vi "Permanentes_Aux.vi"() -> ()   [LabVIEW 2013]
uses:
  <vilib>/Utility/miscctls.llb/LVStringsAndValuesArrayTypeDef_U16.ctl
panel:
  in  "Puerto COM":refnum<visa-resource-name>
  out "Recetas":T1
  in  "Programa":u16(ring)
  in  "Recetas Allen Bradley":T2(array[cluster]) {"Parámetros Modbus"."Acción al desconectar" items=["Alarmar"=0, "Nada"=3]; "Parámetros Modbus"."Timeout" format="%#_g seg."; "Parámetros Modbus"."Formato de mensaje" items=["8-N-1", "8-E-1", "8-O-1", "8-N-2", "8-E-2", "8-O-2"]; "Parámetros Modbus"."Velocidad" items=["1200 baudios", "2400 baudios", "4800 baudios", "9600 baudios", "19200 baudios", "38400 baudios"]; "Parámetros Modbus"."Identificador" min=1 max=255; "Parámetros Modbus"."Frecuencia estándar" format="%.0fHz."; "Características del motor"."Frecuencia máxima" max=500 format="%.0f Hz."; "Características del motor"."Frecuencia mínima" max=500 format="%.0f Hz."; "Características del motor"."Desaceleración" format="%#_g seg."; "Características del motor"."Aceleración" format="%#_g seg."; "Características del motor"."Velocidad nomial" min=0.0 max=24000.0 format="%#_g rpm"; "Características del motor"."Número de polos" min=2 max=40 format="%.0f polos"; "Características del motor"."Corriente nominal" format="%#_g Amp."; "Características del motor"."Corriente sobrecarga" format="%#_g Amp."; "Características del motor"."Frecuencia nominal" min=15 max=500 format="%.0f Hz."; "Características del motor"."Voltaje nominal" min=20.0 max=440.0 format="%#_g V"; "I/O"."Relevador (R)" items=["Listo/Fallo"=0, "Modbus"=13]; "I/O"."Entrada 6 (06)" items=["Sin asignar"=0, "Fallo auxiliar"=12, "Reset"=13]; "I/O"."Entrada 5 (05)" items=["Sin asignar"=0, "Fallo auxiliar"=12, "Reset"=13]; "I/O"."Entrada 3 (03)" items=["Sin asignar"=0, "Fallo auxiliar"=12, "Reset"=13, "2 hilos REV"=50, "3 hilos DIR"=51]; "I/O"."Entrada 2 (02)" items=["Sin asignar"=0, "Fallo auxiliar"=12, "Reset"=13, "2 hilos FWD"=48, "3 hilos RUN"=49]; "Referencias"."Referencia de frecuencia 2" items=["Potenciómetro"=0, "Modbus"=2]; "Referencias"."Referencia de arranque 2" items=["Teclado", "Pulso", "Modbus"]; "Referencias"."Referencia de frecuencia 1" items=["Potenciómetro"=0, "Modbus"=2]; "Referencias"."Referencia de arranque 1" items=["Teclado", "Pulso", "Modbus"]}
  in  "Recetas Schneider":T3(array[cluster]) {"Parámetros Modbus"."Acción al desconectar" items=["Nada", "Alarmar"]; "Parámetros Modbus"."Timeout" format="%#_g seg."; "Parámetros Modbus"."Formato de mensaje" items=["No", "Auto", "8-O-1", "8-E-1", "8-N-1", "8-N-2", "7-O-1", "7-E-1", "7-O-2", "7-E-2"]; "Parámetros Modbus"."Velocidad" items=["No"=0, "4800 baudios"=24, "9600 baudios"=28, "19200 baudios"=32, "38400 baudios"=36]; "Parámetros Modbus"."Identificador" min=1 max=255; "Parámetros Modbus"."Frecuencia estándar" format="%.0fHz."; "Características del motor"."Desaceleración" format="%#_g seg."; "Características del motor"."Aceleración" format="%#_g seg."; "Características del motor"."Frecuencia máxima" format="%#_g Hz."; "Características del motor"."Velocidad nominal" format="%.0f rpm"; "Características del motor"."Frecuencia nominal" format="%#_g Hz."; "Características del motor"."Corriente nominal" format="%#_g Amp."; "Características del motor"."Voltaje nominal" format="%.0f V"; "Características del motor"."Potencia nominal" format="%#_g HP"; "Características del motor"."Frecuencia estándar" items=["50 Hz.", "60 Hz."]; "I/O"."Transistor (DQ)" items=["Modbus", "Sin Fallo", "Run", "Frecuencia alcanzada", "V. Máx. Alcanzada"]; "I/O"."Relevador 2" items=["Modbus", "Sin Fallo", "Run", "Frecuencia alcanzada", "V. Máx. Alcanzada"]; "I/O"."Relevador 1" items=["Modbus", "Sin Fallo", "Run", "Frecuencia alcanzada", "V. Máx. Alcanzada"]; "I/O"."Entrada 6 (DI6)" items=["Sin asignar"=0, "Marcha"=1, "Marcha av."=2, "Marcha atr."=3, "Referencia 1 Fr."=96, "Referencia 2 Fr."=97, "Referencia 1 Run"=98, "Referencia 2 Run"=99]; "I/O"."Entrada 5 (DI5)" items=["Sin asignar"=0, "Marcha"=1, "Marcha av."=2, "Marcha atr."=3, "Referencia 1 Fr."=96, "Referencia 2 Fr."=97, "Referencia 1 Run"=98, "Referencia 2 Run"=99]; "I/O"."Entrada 4 (DI4)" items=["Sin asignar"=0, "Marcha"=1, "Marcha av."=2, "Marcha atr."=3, "Referencia 1 Fr."=96, "Referencia 2 Fr."=97, "Referencia 1 Run"=98, "Referencia 2 Run"=99]; "I/O"."Entrada 3 (DI3)" items=["Sin asignar"=0, "Marcha"=1, "Marcha av."=2, "Marcha atr."=3, "Referencia 1 Fr."=96, "Referencia 2 Fr."=97, "Referencia 1 Run"=98, "Referencia 2 Run"=99]; "I/O"."Entrada 2 (DI2)" items=["Sin asignar"=0, "Marcha"=1, "Marcha av."=30, "Marcha atr."=31, "Referencia 1 Fr."=96, "Referencia 2 Fr."=97, "Referencia 1 Run"=98, "Referencia 2 Run"=99]; "I/O"."Entrada 1 (DI1)" items=["Sin asignar"=0, "Marcha"=1, "Marcha av."=30, "Marcha atr."=31, "Referencia 1 Fr."=96, "Referencia 2 Fr."=97, "Referencia 1 Run"=98, "Referencia 2 Run"=99]; "Referencias"."Referencia de frecuencia 2" items=["No"=0, "Modbus"=164, "Potenciómetro"=183]; "Referencias"."Referencia de arranque 2" items=["Pulso"=0, "Modbus"=9]; "Referencias"."Referencia de frecuencia 1" items=["No"=0, "Modbus"=164, "Potenciómetro"=183]; "Referencias"."Referencia de arranque 1" items=["Pulso"=0, "Modbus"=9]}
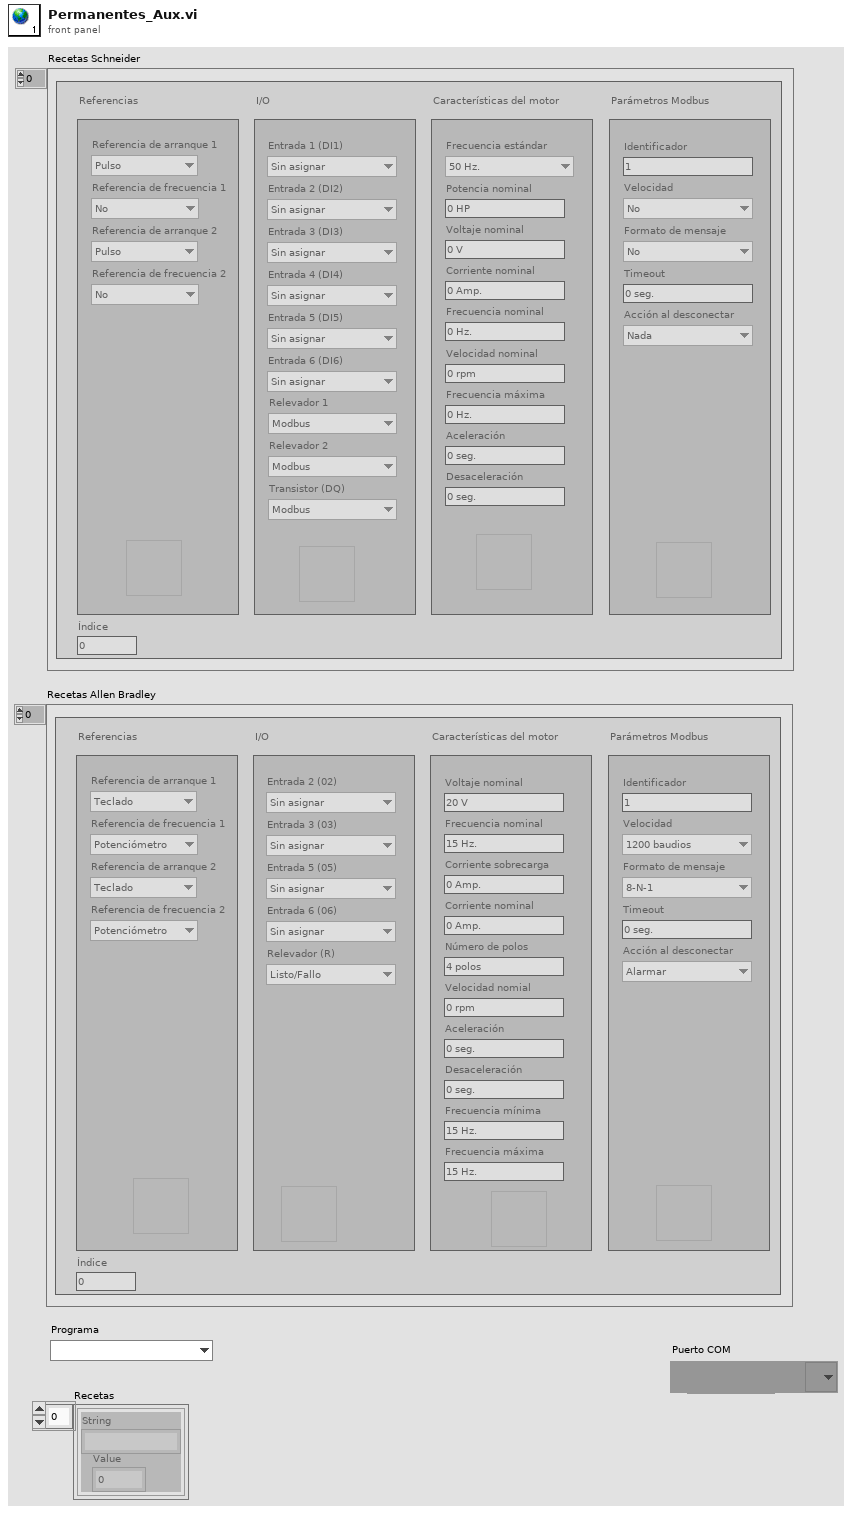
[diagram p1: front panel]
types:
  T1 = typedef "LVStringsAndValuesArrayTypeDef_U16.ctl" = cluster{"String":string, "Value":u16}[]
  T2 = cluster{"Referencias":cluster{"Referencia de arranque 1":u16, "Referencia de frecuencia 1":u16, "Referencia de arranque 2":u16, "Referencia de frecuencia 2":u16, "Configurar":bool}, "I/O":cluster{"Entrada 2 (02)":u16, "Entrada 3 (03)":u16, "Entrada 5 (05)":u16, "Entrada 6 (06)":u16, "Relevador (R)":u16, "Configurar":bool}, "Características del motor":cluster{"Voltaje nominal":dbl, "Frecuencia nominal":u16, "Corriente sobrecarga":dbl, "Corriente nominal":dbl, "Número de polos":u16, "Velocidad nomial":dbl, "Aceleración":dbl, "Desaceleración":dbl, "Frecuencia mínima":u16, "Frecuencia máxima":u16, "Configurar":bool}, "Parámetros Modbus":cluster{"Frecuencia estándar":i32, "Identificador":u16, "Velocidad":u16, "Formato de mensaje":u16, "Timeout":dbl, "Acción al desconectar":u16, "Configurar":bool}, "Índice":i32}[]
  T3 = cluster{"Referencias":cluster{"Referencia de arranque 1":u16, "Referencia de frecuencia 1":u16, "Referencia de arranque 2":u16, "Referencia de frecuencia 2":u16, "Configurar":bool}, "I/O":cluster{"Entrada 1 (DI1)":u16, "Entrada 2 (DI2)":u16, "Entrada 3 (DI3)":u16, "Entrada 4 (DI4)":u16, "Entrada 5 (DI5)":u16, "Entrada 6 (DI6)":u16, "Relevador 1":u16, "Relevador 2":u16, "Transistor (DQ)":u16, "Configurar":bool}, "Características del motor":cluster{"Frecuencia estándar":u16, "Potencia nominal":dbl, "Voltaje nominal":u16, "Corriente nominal":dbl, "Frecuencia nominal":dbl, "Velocidad nominal":u16, "Frecuencia máxima":dbl, "Aceleración":dbl, "Desaceleración":dbl, "Configurar":bool}, "Parámetros Modbus":cluster{"Frecuencia estándar":i32, "Identificador":u16, "Velocidad":u16, "Formato de mensaje":u16, "Timeout":dbl, "Acción al desconectar":u16, "Configurar":bool}, "Índice":i32}[]
diagram:
